vi "Multiple injection_test.vi"() -> ()   [LabVIEW 2020]
uses:
  <vilib>/Powertrain Controls/Device Drivers/Engine Position Tracking/EPTx/RevA/FPGA/Extras/Command Sequence - 8e.vi
  <vilib>/Powertrain Controls/Device Drivers/Engine Position Tracking/EPTx/RevA/FPGA/EPTx - RevA - FPGA.lvlib
panel:
  out "波形图表":i16(graph)
  in  "GlobalTrigger":bool
  in  "SeqReset":bool
  out "Cmd":bool
  out "Paused":bool=TRUE
  out "CmdTimer":u32
  out "SeqPointer":u8
  in  "ContinueSeq8":bool
  in  "ContinueSeq7":bool=TRUE
  in  "ContinueSeq6":bool=TRUE
  in  "ContinueSeq5":bool=TRUE
  in  "ContinueSeq4":bool=TRUE
  in  "ContinueSeq3":bool=TRUE
  in  "ContinueSeq2":bool=TRUE
  in  "ContinueSeq1":bool=TRUE
  in  "CmdLevelSeq8":bool
  in  "CmdLevelSeq7":bool=TRUE
  in  "CmdLevelSeq6":bool
  in  "CmdLevelSeq5":bool=TRUE
  in  "CmdLevelSeq4":bool
  in  "CmdLevelSeq3":bool=TRUE
  in  "CmdLevelSeq2":bool
  in  "CmdLevelSeq1":bool=TRUE
  in  "DurationSeq8":u32=2
  in  "DurationSeq7":u32=2
  in  "DurationSeq6":u32=4
  in  "DurationSeq5":u32=16
  in  "DurationSeq4":u32=4
  in  "DurationSeq3":u32=2
  in  "DurationSeq2":u32=4
  in  "DurationSeq1":u32=2
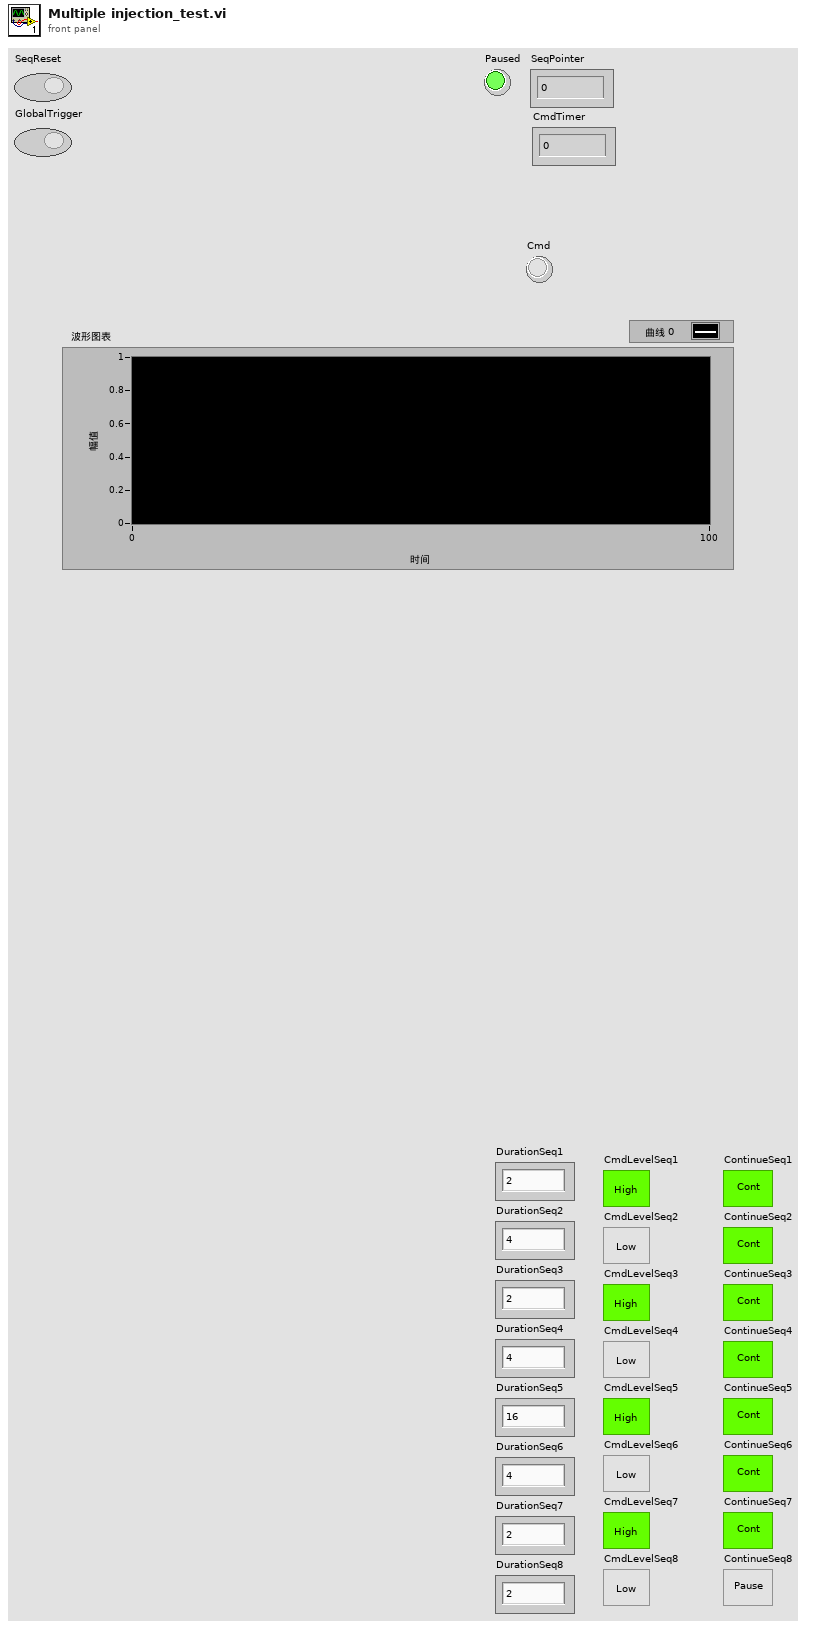
[diagram p1: front panel]
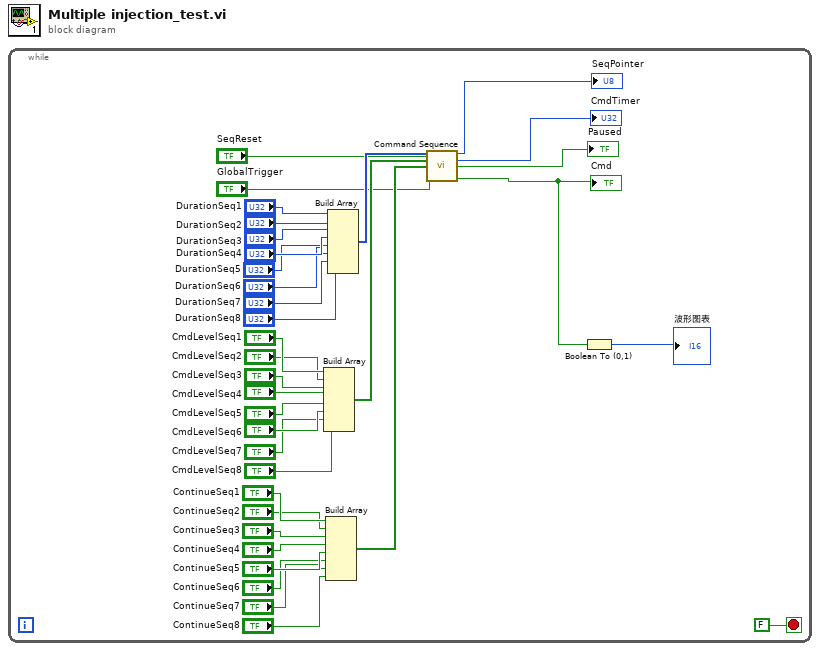
[diagram p0: block diagram]
diagram:
  n1 = while {
    stop <- FALSE stop-if-true
    n2 = Build Array("CmdLevelSeq1", "CmdLevelSeq2", "CmdLevelSeq3", "CmdLevelSeq4", "CmdLevelSeq5", "CmdLevelSeq6", "CmdLevelSeq7", "CmdLevelSeq8") -> (w10:bool[])
    n3 = Build Array("ContinueSeq1", "ContinueSeq2", "ContinueSeq3", "ContinueSeq4", "ContinueSeq5", "ContinueSeq6", "ContinueSeq7", "ContinueSeq8") -> (w9:bool[])
    n4 = Build Array("DurationSeq1", "DurationSeq2", "DurationSeq3", "DurationSeq4", "DurationSeq5", "DurationSeq6", "DurationSeq7", "DurationSeq8") -> (w27:u32[])
    n5 = call-poly <vilib>:"Command Sequence.vi"("DurationSeq"=w27, "CmdLevelSeq"=w10, "ContinueSeq"=w9, "SeqReset"="SeqReset", "GlobalTrigger"="GlobalTrigger") -> ("SeqPointer"=→"SeqPointer":u8, "CmdTimer"=→"CmdTimer":u32, "Paused"=→"Paused":bool, "Cmd"=w2:bool)  [unwired: 7 in]
    "Cmd" <- w2
    n6 = Boolean To (0,1)(Boolean=w2) -> (0, 1=→"波形图表":i16)
  }
